vi "click.vi"(7 "page":i32, 9 "Coords":T1, 10 "Cluster":cluster{"left":i16, "top":i16}, 11 "size":i32) -> (1 "y":i32, 2 "x":i32)   [LabVIEW 2025]
uses:
  <vilib>/Utility/miscctls.llb/LVPoint32TypeDef.ctl
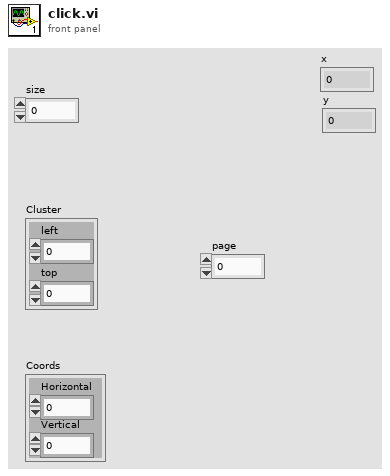
[diagram p1: front panel]
types:
  T1 = typedef "LVPoint32TypeDef.ctl" = cluster{"Horizontal":i32, "Vertical":i32}
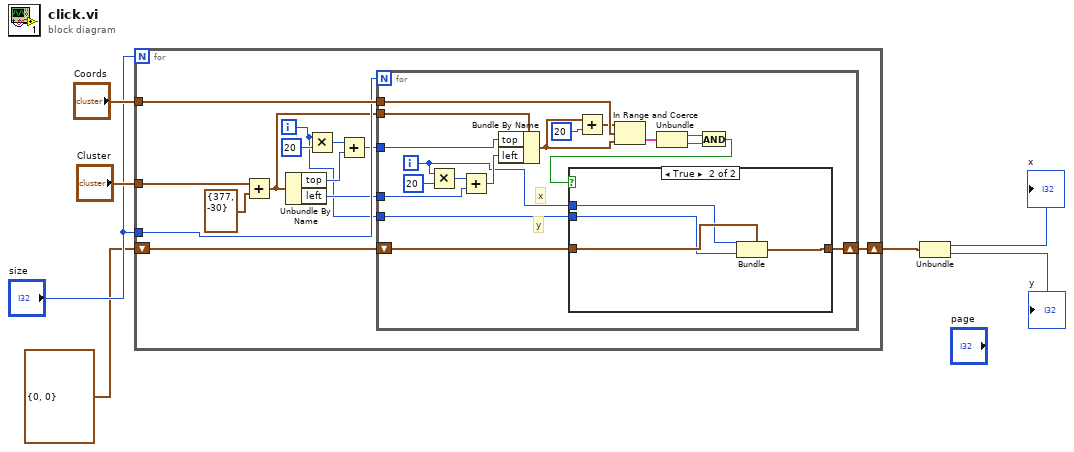
[diagram p0: block diagram]
diagram:
  n1 = for {
    N: "size" -> [_]
    tunnel: "Cluster" -> [w12]
    tunnel: "Coords" -> [w20]
    tunnel: "size" -> [w19]
    shift-right: [w9] -> w3
    shift-left: cluster{i32, i32} {0, 0} -> [w10]
    i -> [w8]
    n2 = Add(x=w12, y=cluster{"left":i16, "top":i16} {"left"=377, "top"=-30}) -> (x+y=w11:cluster{"left":i16, "top":i16})
    n3 = Unbundle By Name(w11) -> ("top"=w18:i16, "left"=w14:i16)
    n4 = Multiply(x=w8, y=i16 20 ("x")) -> (x*y=w16:i32)
    n5 = Add(x=w16, y=w18) -> (x+y=w15:i32)
    n6 = for {
      N: w19 -> [_]
      tunnel: w20 -> [w38]
      tunnel: w15 -> [w34]
      tunnel: w14 -> [w35]
      tunnel: w11 -> [w32]
      shift-right: [w23] -> w9
      shift-left: w10 -> [w24]
      tunnel: w8 -> [w22]
      i -> [w21]
      # "y"
      # "x"
      n7 = Multiply(x=w21, y=i16 20 ("x")) -> (x*y=w36:i32)
      n8 = Add(x=w36, y=w35) -> (x+y=w33:i32)
      n9 = Bundle By Name(cluster=w32, "top"=w34, "left"=w33) -> (w29:cluster{"left":i16, "top":i16})
      n10 = Add(x=w29, y=i16 20 ("x")) -> (x+y=w30:cluster{"left":i16, "top":i16})
      n11 = In Range and Coerce(upper limit=w30, x=w38, lower limit=w29) -> (In Range?=w28:cluster{"Horizontal":bool, "Vertical":bool})  [unwired: 1 out]
      n12 = Unbundle(w28) -> ("Horizontal"=w27:bool, "Vertical"=w26:bool)
      n13 = And(x=w27, y=w26) -> (x .and. y?=w25:bool)
      n14 = case shown="True" w25 {
        tunnel: [w39 w40] -> w23
        tunnel: w24 -> [w39 w43]
        tunnel: w22 -> [_ w41]
        tunnel: w21 -> [_ w42]
        frame False {
        }
        frame True {
          n15 = Bundle(cluster=w43, w42, w41) -> (w40:cluster{i32, i32})
        }
      }
    }
  }
  n16 = Unbundle(w3) -> (→"x":i32, →"y":i32)
